vi "Get Tx Acyclic Message Configuration.vi"(8 "error in":errorcluster, 10 "configuration string":string, 11 "port":T1 format="%.0x") -> (0 "error out":errorcluster, 2 "configuration string out":string, 3 "port out":T1 format="%.0x")   [LabVIEW 2020, in "Ballard ARINC 429 Hardware Configuration.lvlib"]
uses:
  Ballard ARINC 429 Hardware Configuration.lvlib
  <vilib>/NI VeriStand/Custom Device API/Custom Device Item Ref.ctl
  Constants.vi
  Scripting/Ballard/Ballard ARINC 429 Scripting.lvlib
  Scripting/ARINC 429/ARINC 429 Scripting.lvlib
  <vilib>/NI VeriStand/Custom Device API/Custom Device API.lvlib
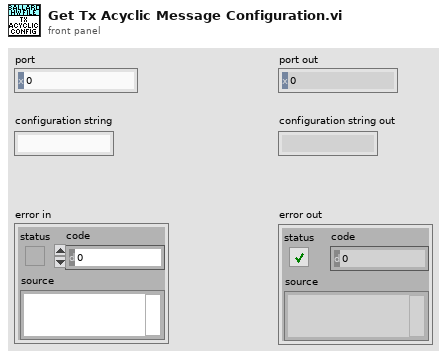
[diagram p1: front panel]
types:
  T1 = typedef "Custom Device API.lvlib/Custom Device Item Ref.ctl" = u64
  T2 = typedef "Label Properties.ctl" = cluster{"label (Dec)":T3, "SDI value":u8, "SDI enabled":bool}
  T3 = typedef "Label.ctl" = u8
  T4 = typedef "Transfer Type.ctl" = enum16{"Scheduled", "Acyclic", "Block", "Strobe"}
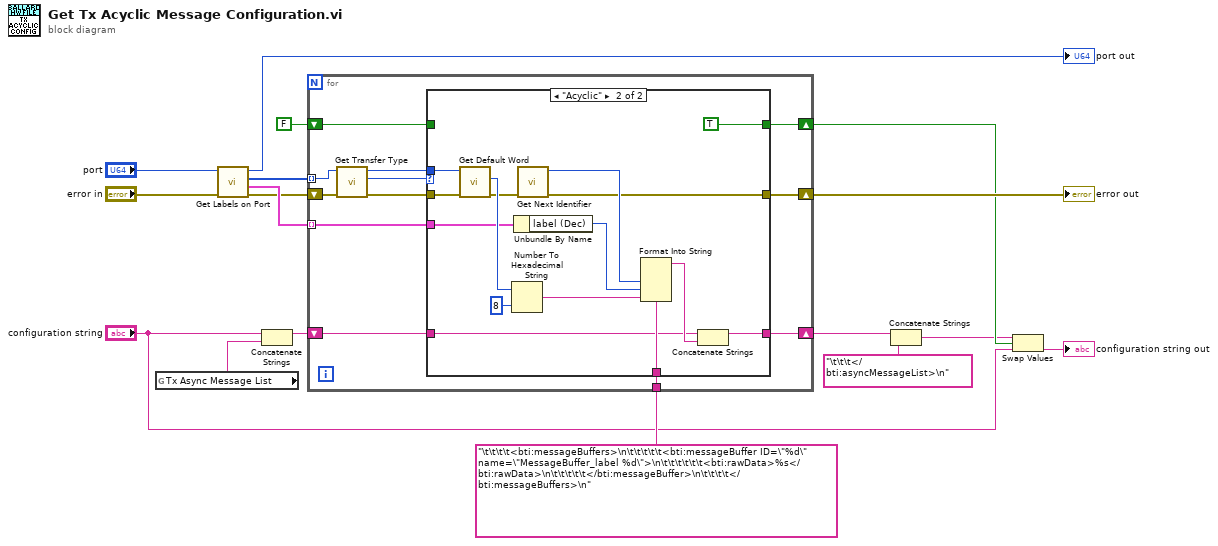
[diagram p0: block diagram]
diagram:
  n1 = global read "Constants.vi" "Tx Async Message List"() -> (w1:string)
  n2 = call "Get Labels on Port.vi"("error in"="error in", "port in"="port") -> ("error out"=w10:errorcluster, "labels properties"=w13:T2[], "labels"=w12:T1[], "port out"=→"port out":T1)  [unwired: 6 in]
  n3 = Concatenate Strings("configuration string", w1) -> (w14:string)
  n4 = for {
    shift-right: [w26] -> w5
    shift-left: w14 -> [w27]
    tunnel: w13 -> [w28] mode=indexing
    tunnel: w12 -> [w22] mode=indexing
    tunnel: "\t\t\t\t<bti:messageBuffers>\n\t\t\t\t\t<bti:messageBuffer ID=\"%d\" name=\"MessageBuffer_label %d\">\n\t\t\t\t\t\t<bti:rawData>%s</bti:rawData>\n\t\t\t\t\t</bti:messageBuffer>\n\t\t\t\t</bti:messageBuffers>\n" -> [w29]
    shift-right: [w25] -> w9
    shift-left: w10 -> [w24]
    shift-right: [w18] -> w6
    shift-left: FALSE -> [w19]
    n5 = call "Get Transfer Type.vi"("error in"=w24, "label ref in"=w22) -> ("error out"=w23:errorcluster, "transfer type"=w20:T4, "label ref out"=w21:T1)  [unwired: 7 in]
    n6 = case shown="\"Acyclic\"" w20 {
      tunnel: w29 -> [_ w47]
      tunnel: w28 -> [_ w40]
      tunnel: w27 -> [w31 w42]
      tunnel: [w31 w41] -> w26
      tunnel: [w32 w33] -> w25
      tunnel: w23 -> [w32 w36]
      tunnel: w21 -> [_ w35]
      tunnel: w19 -> [w30 _]
      tunnel: [w30 TRUE] -> w18
      frame Default {
      }
      frame "Acyclic" {
        n7 = call "Get Default Word.vi"("error in"=w36, "Item Ref in"=w35) -> ("error out"=w34:errorcluster, "default word"=w45:u32)  [unwired: 7 in, 1 out]
        n8 = Number To Hexadecimal String(1:i16 8 ("width (-)"), 2:w45) -> (0:w38:string)
        n9 = Unbundle By Name(w40) -> ("label (Dec)"=w39:T3)
        n10 = call "Get Next Identifier.vi"("error in"=w34) -> ("error out"=w33:errorcluster, "ID"=w46:u32)  [unwired: 9 in]
        n11 = Format Into String(format string=w47, w46, w39, w38) -> (resulting string=w43:string)  [unwired: 2 in, 1 out]
        n12 = Concatenate Strings(w42, w43) -> (w41:string)
      }
    }
  }
  "error out" <- w9
  n13 = Concatenate Strings(w5, "\t\t\t</bti:asyncMessageList>\n") -> (w4:string)
  n14 = Swap Values(12:w4, 13:w6, 14:"configuration string") -> (3:→"configuration string out":string)  [unwired: 1 out]
